vi "Write Multiple Coils.vi"(8 "error in (no error)":errorcluster, 9 "coil values":bool[](array[boolean]), 10 "starting address":u16, 11 "Modbus slave in":refnum<class "Modbus Slave.lvclass">) -> (0 "error out":errorcluster, 3 "Modbus slave out":refnum<class "Modbus Slave.lvclass">)   [LabVIEW 2015, in "Modbus Slave.lvclass"]
doc: "Writes values to contiguous coils."
uses:
  <vilib>/Modbus/slave/Modbus Slave.lvclass
  <vilib>/Modbus/slave/Modbus Slave.lvclass/Modbus Slave.ctl
  <vilib>/Modbus/subvis/Data and Functions/Device Data Model/Device Data Model.lvclass
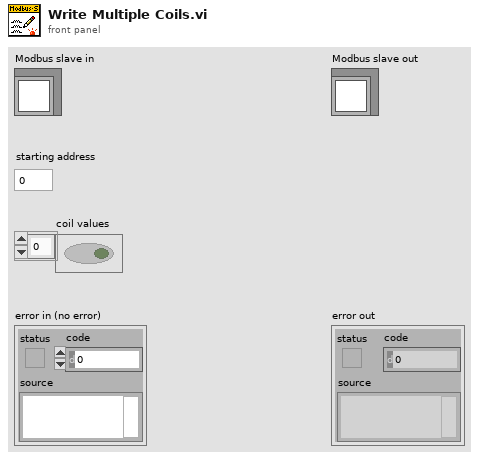
[diagram p1: front panel]
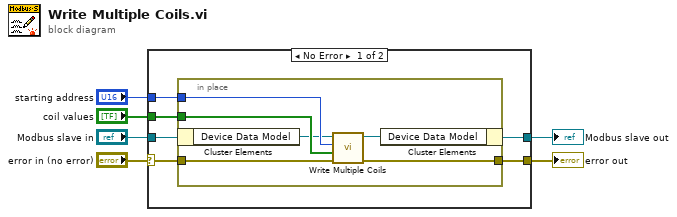
[diagram p0: block diagram]
diagram:
  n1 = case shown="No Error" "error in (no error)" {
    selector: "error in (no error)" -> [w8 w20]
    tunnel: [w7 w20] -> w3
    tunnel: "Modbus slave in" -> [w10 w19]
    tunnel: "coil values" -> [w12 _]
    tunnel: "starting address" -> [w11 _]
    tunnel: [w9 w19] -> w1
    frame No Error {
      n2 = in-place {
        in-place-border: [w18] -> w7
        in-place-border: w12 -> [w17]
        in-place-border: w11 -> [w16]
        in-place-border: w8 -> [w13]
        n3 = in-place-cluster #1(w10) -> ("Device Data Model"=w14:refnum<class "Device Data Model.lvclass">)
        n4 = call-dynamic "Write Multiple Coils.vi"("error in (no error)"=w13, "coils"=w17, "starting address"=w16, "device data model in"=w14) -> ("error out"=w18:errorcluster, "device data model out"=w15:refnum<class "Device Data Model.lvclass">)  [unwired: 6 in]
        n5 = in-place-cluster #1("Device Data Model"=w15) -> (w9:refnum<class "Modbus Slave.lvclass">)
      }
    }
    frame Error {
    }
  }
  "error out" <- w3
  "Modbus slave out" <- w1
